vi "Compression_Simulation.vi"(5 "measure call context in":refnum<class "Measure Call Context.lvclass">, 7 "SMU Settings":T2={"SMU Name"="PXI1Slot15", "SMU Channel"="2"}, 8 "error in":errorcluster, 11 "Test Configuration":T3={"Expected DUT Gain (dB)"=17.5, "Max Linear Range (dBm)"=-10.0, "Compression Point (dB)"=1.0, "Pout at Pin (dBm)"=1.0, "RFSG Frequency Start (Hz)"=6000000000.0, "RFSG Frequency Stop (Hz)"=18000000000.0, "RFSG Number of Frequency Step"=10, "Power Start (dBm)"=-20.0, "Power Stop(dBm)"=1.0, "Power Step Size (dB)"=4.0, "RBW (Hz)"=5000000.0} {"Pout at Pin (dBm)" format="%#pdBm"; "RFSG Frequency Stop (Hz)" format="%#_6p"; "Power Start (dBm)" format="%#_6p"; "Power Stop(dBm)" format="%#_6p"; "RFSG Frequency Start (Hz)" format="%#_6p"; "Expected DUT Gain (dB)" step=1.0 format="%#_6p"}) -> (0 "error out":errorcluster, 3 "Data":T1)   [LabVIEW 2023]
doc: "This example demonstrates how to use MMICsc API for performing PAE measurements and calibration"
uses:
  Controls/Test Config - Compression.ctl
  <vilib>/Plug-In SDKs/Measurements/Measure Call Context/Measure Call Context.lvclass
  Controls/SMU Config - Compression.ctl
  Controls/Results - Compression.ctl
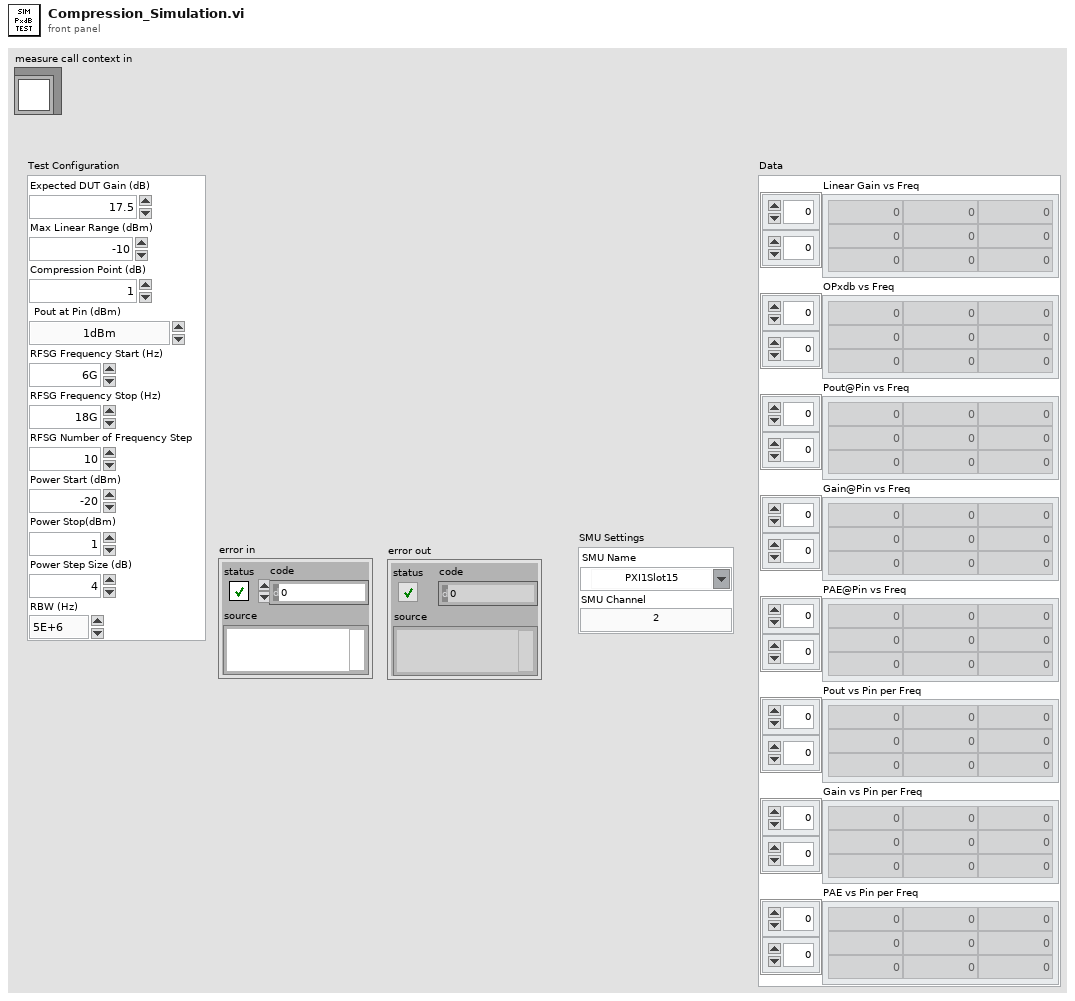
[diagram p1: front panel]
types:
  T1 = typedef "Results - Compression.ctl" = cluster{"Linear Gain vs Freq":dbl[][], "OPxdb vs Freq":dbl[][], "Pout@Pin vs Freq":dbl[][], "Gain@Pin vs Freq":dbl[][], "PAE@Pin vs Freq":dbl[][], "Pout vs Pin per Freq":dbl[][], "Gain vs Pin per Freq":dbl[][], "PAE vs Pin per Freq":dbl[][]}
  T2 = typedef "SMU Config - Compression.ctl" = cluster{"SMU Name":refnum<k15>, "SMU Channel":string}
  T3 = typedef "Test Config - Compression.ctl" = cluster{"Expected DUT Gain (dB)":dbl, "Max Linear Range (dBm)":dbl, "Compression Point (dB)":dbl, "Pout at Pin (dBm)":dbl, "RFSG Frequency Start (Hz)":dbl, "RFSG Frequency Stop (Hz)":dbl, "RFSG Number of Frequency Step":i32, "Power Start (dBm)":dbl, "Power Stop(dBm)":dbl, "Power Step Size (dB)":dbl, "RBW (Hz)":dbl}
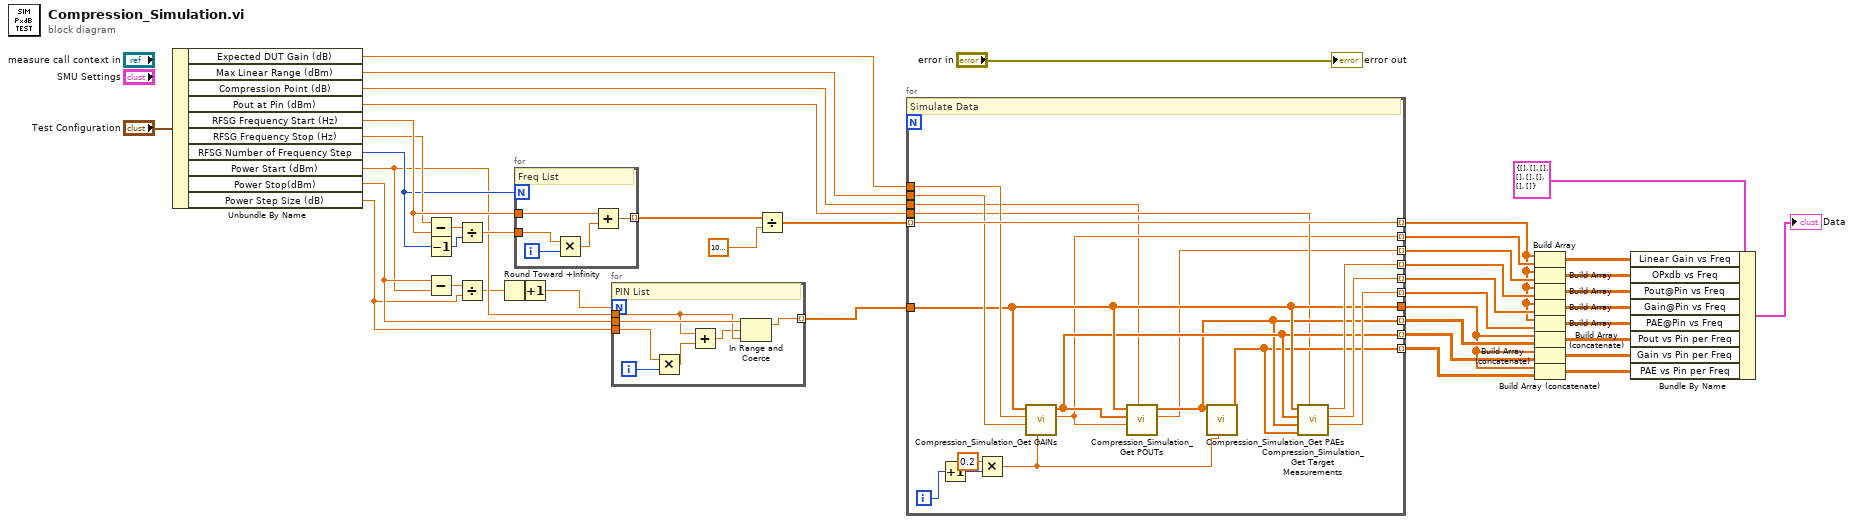
[diagram p0: block diagram]
diagram:
  n1 = Unbundle By Name("Test Configuration") -> ("Expected DUT Gain (dB)"=w29:dbl, "Max Linear Range (dBm)"=w30:dbl, "Compression Point (dB)"=w28:dbl, "Pout at Pin (dBm)"=w10:dbl, "RFSG Frequency Start (Hz)"=w42:dbl, "RFSG Frequency Stop (Hz)"=w41:dbl, "RFSG Number of Frequency Step"=w38:i32, "Power Start (dBm)"=w35:dbl, "Power Stop(dBm)"=w36:dbl, "Power Step Size (dB)"=w33:dbl)
  n2 = Subtract(x=w41, y=w42) -> (x-y=w40:dbl)
  n3 = Decrement(x=w38) -> (x-1=w37:i32)
  n4 = Subtract(x=w36, y=w35) -> (x-y=w34:dbl)
  n5 = Divide(x=w40, y=w37) -> (x/y=w39:dbl)
  n6 = Divide(x=w34, y=w33) -> (x/y=w32:dbl)
  n7 = Round Toward +Infinity(x=w32) -> (ceil(x): smallest int >= x=w31:dbl)
  n8 = for {
    N: w38 -> [_]
    tunnel: w42 -> [w48]
    tunnel: w39 -> [w45]
    tunnel: [w44] -> w27 mode=indexing
    i -> [w46]
    # "Freq List"
    n9 = Multiply(x=w45, y=w46) -> (x*y=w47:dbl)
    n10 = Add(x=w48, y=w47) -> (x+y=w44:dbl)
  }
  n11 = Increment(x=w31) -> (x+1=w21:dbl)
  n12 = for {
    N: w21 -> [_]
    tunnel: w35 -> [w53]
    tunnel: [w55] -> w20 mode=indexing
    tunnel: w36 -> [w54]
    tunnel: w33 -> [w49]
    i -> [w51]
    # "PIN List"
    n13 = Multiply(x=w49, y=w51) -> (x*y=w50:dbl)
    n14 = Add(x=w53, y=w50) -> (x+y=w52:dbl)
    n15 = In Range and Coerce(upper limit=w54, x=w52, lower limit=w53) -> (coerced(x)=w55:dbl)  [unwired: 1 out]
  }
  n16 = Divide(x=w27, y=1000000000.0) -> (x/y=w6:dbl[])
  n17 = for {
    tunnel: w30 -> [w65]
    tunnel: w29 -> [w66]
    tunnel: w28 -> [w58]
    tunnel: w6 -> [w73] mode=indexing
    tunnel: [w73] -> w11 mode=indexing
    tunnel: [w59] -> w26 mode=indexing
    tunnel: [w57] -> w23 mode=indexing
    tunnel: w20 -> [w64]
    tunnel: [w64] -> w9
    tunnel: [w62] -> w19 mode=indexing
    tunnel: [w63] -> w18 mode=indexing
    tunnel: [w72] -> w14 mode=indexing
    tunnel: [w71] -> w13 mode=indexing
    tunnel: [w70] -> w12 mode=indexing
    tunnel: w10 -> [w60]
    tunnel: [w61] -> w8 mode=indexing
    i -> [w67]
    # "Simulate Data"
    n18 = Increment(x=w67) -> (x+1=w68:i32)
    n19 = Multiply(x=0.2, y=w68) -> (x*y=w56:dbl)
    n20 = call "Compression_Simulation_Get GAINs.vi"("Adjusting Factor"=w56, "Max Linear Range (dBm)"=w65, "Expected DUT Gain (dB)"=w66, "PINs in"=w64) -> ("Linear Gain"=w59:dbl, "GAINs out"=w63:dbl[])  [unwired: 6 in]
    n21 = call "Compression_Simulation_Get POUTs.vi"("PxdB"=w58, "Linear Gain"=w59, "GAINs in"=w63, "PINs in"=w64) -> ("OPxdB"=w57:dbl, "POUTs out"=w62:dbl[])  [unwired: 6 in]
    n22 = call "Compression_Simulation_Get PAEs.vi"("Adjusting Factor"=w56, "POUTs in"=w62) -> ("PAEs out"=w61:dbl[])  [unwired: 9 in]
    n23 = call "Compression_Simulation_Get Target Measurements.vi"("Pout at Pin (dBm)"=w60, "PAEs in"=w61, "POUTs in"=w62, "GAINs in"=w63, "PINs in"=w64) -> ("PAE@Pin"=w70:dbl, "Gain@Pin"=w71:dbl, "Pout@Pin"=w72:dbl)  [unwired: 4 in]
  }
  n24 = Build Array(w11, w26) -> (w24:dbl[][])
  n25 = Build Array(w11, w23) -> (w22:dbl[][])
  n26 = Build Array(w11, w14) -> (w17:dbl[][])
  n27 = Build Array(w11, w13) -> (w16:dbl[][])
  n28 = Build Array(w11, w12) -> (w15:dbl[][])
  n29 = Build Array (concatenate)(w9, w19) -> (w4:dbl[][])
  n30 = Build Array (concatenate)(w9, w18) -> (w3:dbl[][])
  n31 = Build Array (concatenate)(w9, w8) -> (w2:dbl[][])
  n32 = Bundle By Name(cluster=T1 {"Linear Gain vs Freq"=[], "OPxdb vs Freq"=[], "Pout@Pin vs Freq"=[], "Gain@Pin vs Freq"=[], "PAE@Pin vs Freq"=[], "Pout vs Pin per Freq"=[], "Gain vs Pin per Freq"=[], "PAE vs Pin per Freq"=[]} ("Data"), "Linear Gain vs Freq"=w24, "OPxdb vs Freq"=w22, "Pout@Pin vs Freq"=w17, "Gain@Pin vs Freq"=w16, "PAE@Pin vs Freq"=w15, "Pout vs Pin per Freq"=w4, "Gain vs Pin per Freq"=w3, "PAE vs Pin per Freq"=w2) -> (→"Data":T1)
  "error out" <- "error in"
